vi "KISSIA_PARSE_MIDE_FLUJOS.vi"(11 "String":string="Mide Bronkhorst 1, mide Alicats 1,  y pausa 1.0s") -> (1 "Pausa (s)":dbl=1.0, 2 "Mide Alicats":bool=TRUE, 3 "Mide Bronkhorst":bool=TRUE)   [LabVIEW 2017]
panel:
  # "Mide Bronkhorst 1, mide Alicats 0,  y pausa 1.0s"
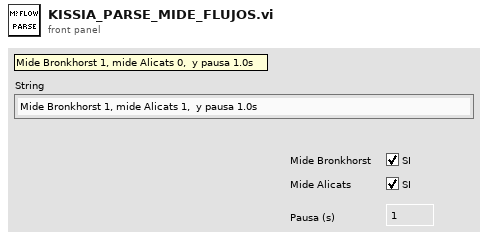
[diagram p1: front panel]
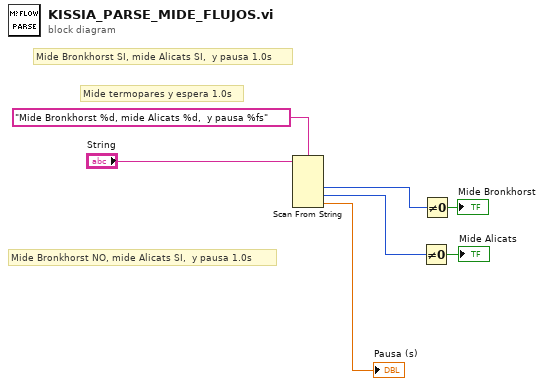
[diagram p0: block diagram]
diagram:
  # "Mide Bronkhorst NO, mide Alicats SI,  y pausa 1.0s"
  # "Mide Bronkhorst SI, mide Alicats SI,  y pausa 1.0s"
  # "Mide termopares y espera 1.0s"
  n1 = Scan From String(format string="Mide Bronkhorst %d, mide Alicats %d,  y pausa %fs", input string="String") -> (output 1=w4:i32, output 2=w1:i32, output 3=→"Pausa (s)":dbl)  [unwired: 5 in, 3 out]
  n2 = Not Equal To 0?(x=w1) -> (x != 0?=→"Mide Alicats":bool)
  n3 = Not Equal To 0?(x=w4) -> (x != 0?=→"Mide Bronkhorst":bool)
